vi "Experiment Serial.vi"() -> ()   [LabVIEW 2009]
panel:
  out "Array":string[](array[string])
  out "read string 2":string
  out "read string":string
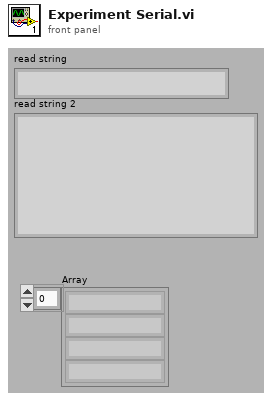
[diagram p1: front panel]
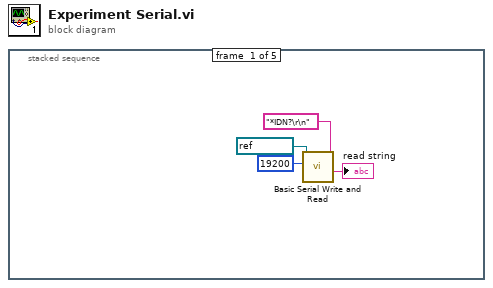
[diagram p0: block diagram]
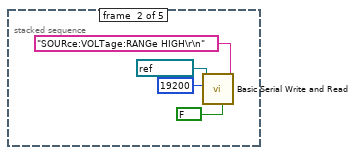
[diagram p2: hidden frame]
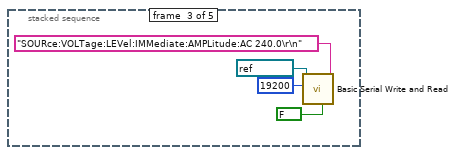
[diagram p3: hidden frame]
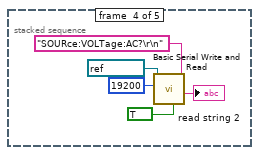
[diagram p4: hidden frame]
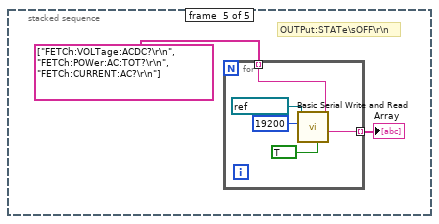
[diagram p5: hidden frame]
diagram:
  n1 = stacked-sequence {
    frame #0 {
      n2 = call "Basic Serial Write and Read.vi"("VISA resource name"=refnum<visa-resource-name> "COM1", "baud rate"=u32 19200, "string to write"="*IDN?\r\n") -> ("read string"=→"read string":string)  [unwired: 6 in, 1 out]
    }
    frame #1 {
      n3 = call "Basic Serial Write and Read.vi"("VISA resource name"=refnum<visa-resource-name> "COM1", "baud rate"=u32 19200, "read"=FALSE, "string to write"="SOURce:VOLTage:RANGe HIGH\r\n") -> ()  [unwired: 5 in, 2 out]
    }
    frame #2 {
      n4 = call "Basic Serial Write and Read.vi"("VISA resource name"=refnum<visa-resource-name> "COM1", "baud rate"=u32 19200, "read"=FALSE, "string to write"="SOURce:VOLTage:LEVel:IMMediate:AMPLitude:AC 240.0\r\n") -> ()  [unwired: 5 in, 2 out]
    }
    frame #3 {
      n5 = call "Basic Serial Write and Read.vi"("VISA resource name"=refnum<visa-resource-name> "COM1", "baud rate"=u32 19200, "read"=TRUE, "string to write"="SOURce:VOLTage:AC?\r\n") -> ("read string"=→"read string 2":string)  [unwired: 5 in, 1 out]
    }
    frame #4 {
      # "OUTPut:STATe\\sOFF\\r\\n"
      n6 = for {
        tunnel: [w21] -> w18 mode=indexing
        tunnel: string[] ["FETCh:VOLTage:ACDC?\r\n", "FETCh:POWer:AC:TOT?\r\n", "FETCh:CURRENT:AC?\r\n"] -> [w20] mode=indexing
        n7 = call "Basic Serial Write and Read.vi"("VISA resource name"=refnum<visa-resource-name> "COM1", "baud rate"=u32 19200, "read"=TRUE, "string to write"=w20) -> ("read string"=w21:string)  [unwired: 5 in, 1 out]
      }
      "Array" <- w18
    }
  }
